vi "MAT Read Matrix.vi"(0 "Ref Num":refnum<file>, 5 "Error In":errorcluster) -> (6 "Matrix Name":string, 8 "Representation":T1, 9 "CSG":csg[][](array[numeric]) format="%.2f", 10 "STR":string[](array[string]), 11 "CDB":cdb[][](array[numeric]) format="%.2f", 12 "DBL":dbl[][](array[numeric]) format="%.2f", 13 "U8":u8[][](array[numeric]), 14 "Dup Ref Num":refnum<file>, 15 "SGL":sgl[][](array[numeric]) format="%.2f", 16 "I32":i32[][](array[numeric]), 17 "I16":i16[][](array[numeric]), 18 "U16":u16[][](array[numeric]), 19 "error out":errorcluster)   [LabVIEW 2013]
doc: "\"Save to MAT\" saves a 2D array of numbers or a 1D array of strings to MATLAB file. It works only with LabVIEW for Windows. All data types, described in MATLAB/External Interface Guide/Appendix A, are supported, except Sparse Matrices.\n\nAll data inputs should be 2D arrays, except String input which should be a 1D array. Only one data input may contain a non-empty array, otherwise error will be generated (error code -1).\n\nSAVML.LLB is a freeware written by Serge Liberman <liber@us1.channel1.com>."
uses:
  MAT Type Representation.ctl
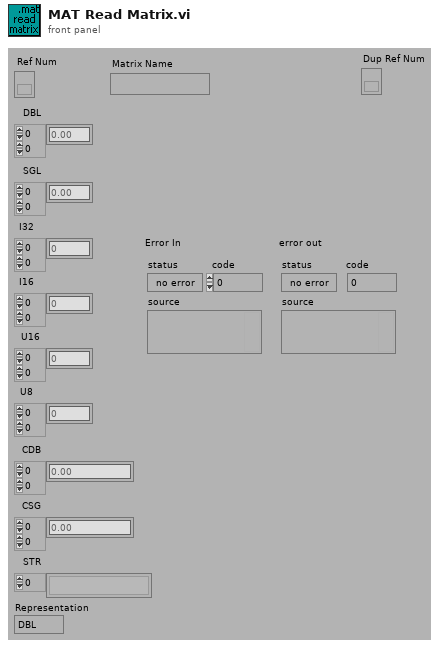
[diagram p1: front panel]
types:
  T1 = typedef "MAT Type Representation.ctl" = enum16{"DBL", "SGL", "I32", "I16", "U16", "U8", "CDB", "CSG", "STR"}
  T2 = enum16{"big-endian, network order", "native, host order", "little-endian"}
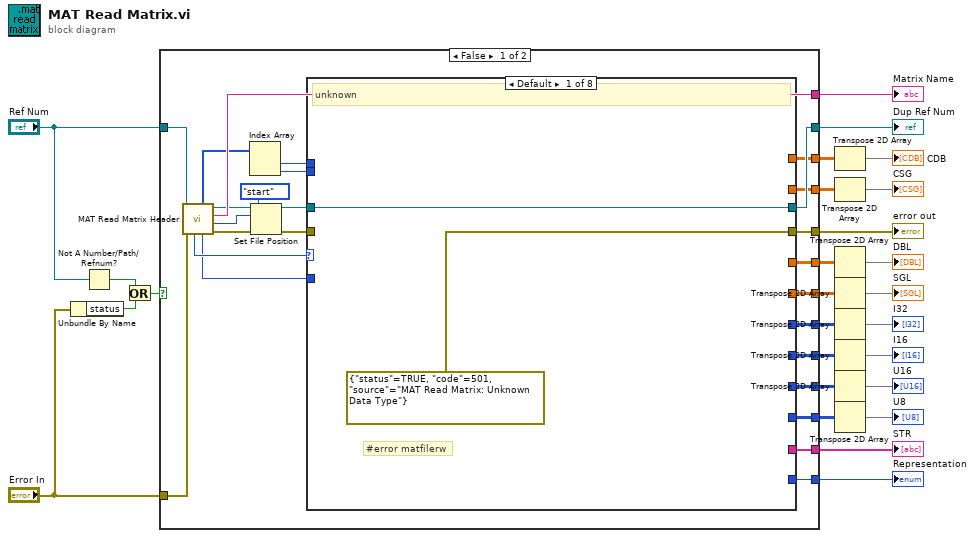
[diagram p0: block diagram]
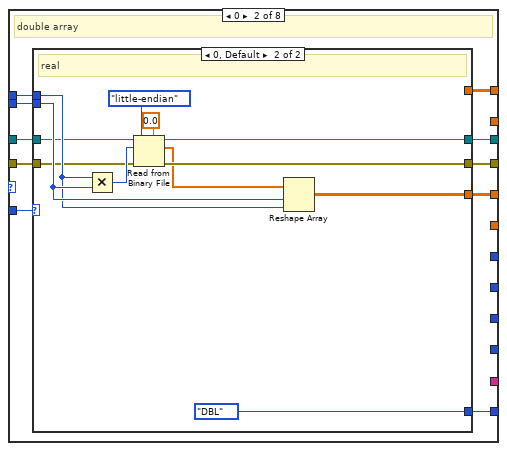
[diagram p2: hidden frame]
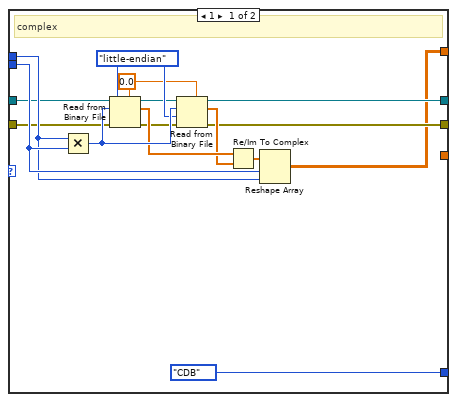
[diagram p3: hidden frame]
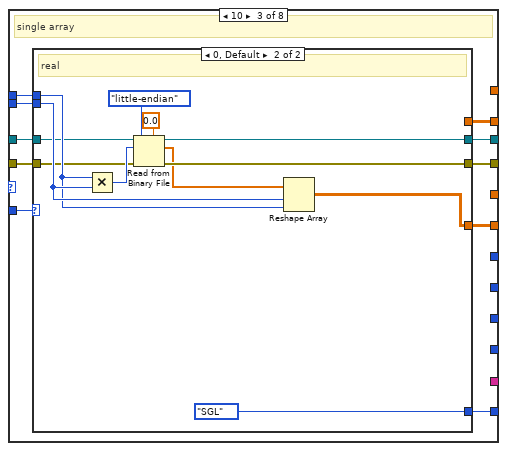
[diagram p4: hidden frame]
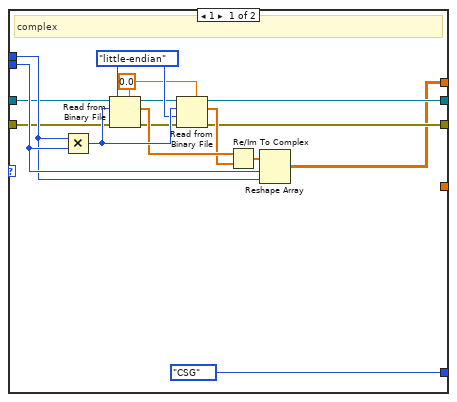
[diagram p5: hidden frame]
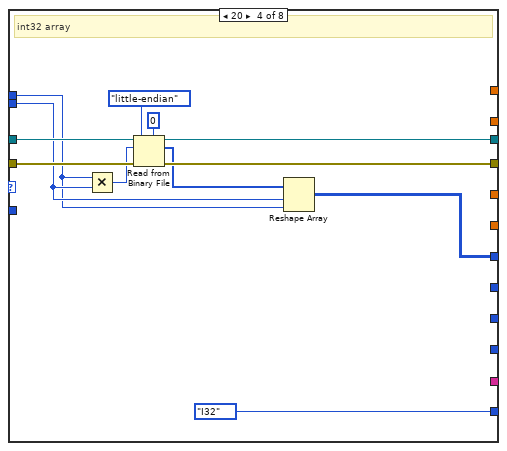
[diagram p6: hidden frame]
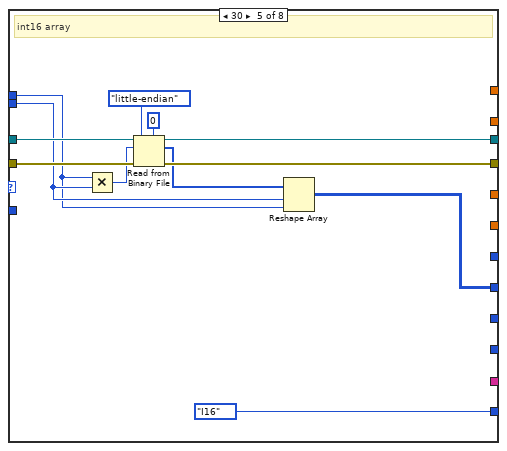
[diagram p7: hidden frame]
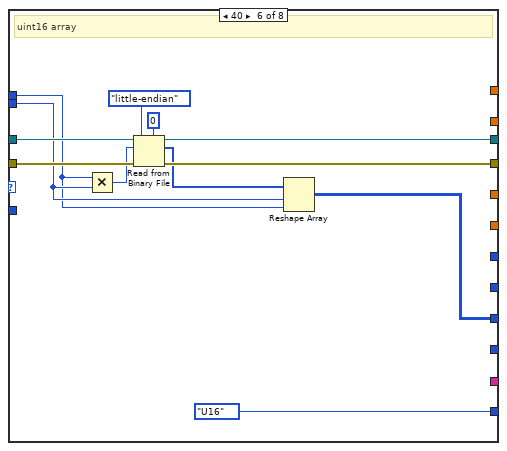
[diagram p8: hidden frame]
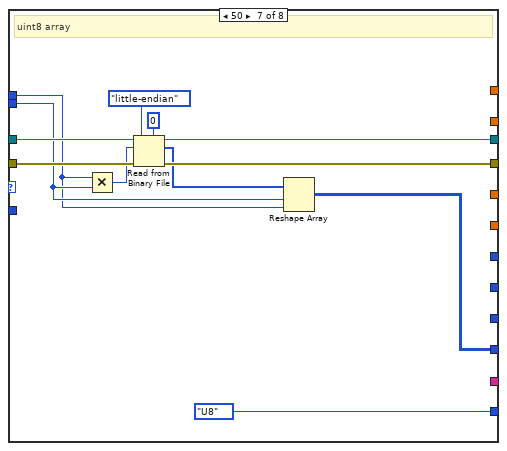
[diagram p9: hidden frame]
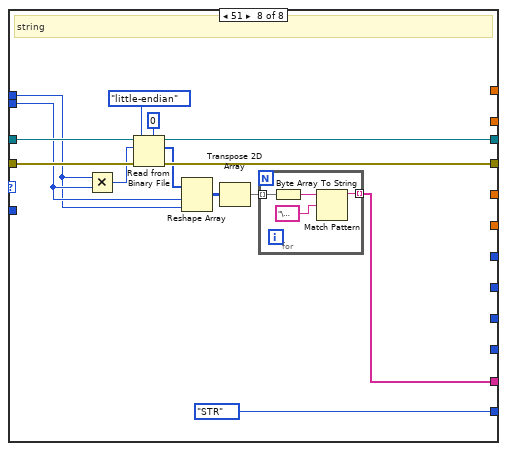
[diagram p10: hidden frame]
diagram:
  n1 = Unbundle By Name("Error In") -> ("status"=w23:bool)
  n2 = Not A Number/Path/Refnum?(number/path/refnum="Ref Num") -> (NaN/Path/Refnum?=w21:bool)
  n3 = Or(x=w21, y=w23) -> (x .or. y?=w20:bool)
  n4 = case shown="False" w20 {
    tunnel: [w52 w198] -> w26
    tunnel: "Ref Num" -> [w50 w198]
    tunnel: "Error In" -> [w36 w197]
    tunnel: [w51 w197] -> w24
    tunnel: [w48 _] -> w19
    tunnel: [w47 _] -> w18
    tunnel: [w46 _] -> w17
    tunnel: [w45 _] -> w16
    tunnel: [w43 _] -> w15
    tunnel: [w42 _] -> w14
    tunnel: [w41 _] -> w13
    tunnel: [w40 _] -> w12
    tunnel: [w39 _] -> w11
    tunnel: [w38 _] -> w3
    tunnel: [w37 _] -> w10
    frame False {
      n5 = call "MAT Read Matrix Header.vi"("Error In"=w36, "Ref Num"=w50) -> ("error out"=w31:errorcluster, "offset"=w29:i32, "Matrix Name"=w48:string, "Dup Ref Num"=w30:refnum<file>, "Real/Complex (0 - Real)"=w44:u32, "Matrix Size (rows x cols)"=w27:i32[], "Rep. Code"=w49:u32)  [unwired: 3 in]
      n6 = Index Array(array=w27) -> (element #1=w34:i32, element #2=w35:i32)  [unwired: 2 in]
      n7 = Set File Position(offset (in bytes) (0)=w29, refnum=w30, from (0:start)=enum16{"start", "end", "current"}."start", error in=w31) -> (refnum out=w32:refnum<file>, error out=w33:errorcluster)
      n8 = case shown="Default" w49 {
        tunnel: w32 -> [w54 w64 w102 w142 w154 w166 w178 w192]
        tunnel: [w54 w63 w101 w141 w153 w165 w177 w191] -> w52
        tunnel: w33 -> [_ w61 w99 w139 w151 w163 w175 w189]
        tunnel: [errorcluster {"status"=TRUE, "code"=501, "source"="MAT Read Matrix: Unknown Data Type"} ("error in (no error)") w62 w100 w140 w152 w164 w176 w190] -> w51
        tunnel: [_ w60 w98 MAT_Type_Representation."I32" ("Representation") MAT_Type_Representation."I16" ("Representation") MAT_Type_Representation."U16" ("Representation") MAT_Type_Representation."U8" ("Representation") MAT_Type_Representation."STR" ("Representation")] -> w47
        tunnel: w35 -> [_ w59 w97 w137 w149 w161 w173 w187]
        tunnel: w34 -> [_ w58 w96 w136 w148 w160 w172 w186]
        tunnel: [_ w57 _ _ _ _ _ _] -> w46
        tunnel: [_ _ w93 _ _ _ _ _] -> w45
        tunnel: w44 -> [_ w56 w95 _ _ _ _ _]
        tunnel: [_ _ _ w131 _ _ _ _] -> w43
        tunnel: [_ _ _ _ w143 _ _ _] -> w42
        tunnel: [_ _ _ _ _ w155 _ _] -> w41
        tunnel: [_ _ _ _ _ _ w167 _] -> w40
        tunnel: [_ _ _ _ _ _ _ w179] -> w39
        tunnel: [_ w55 _ _ _ _ _ _] -> w38
        tunnel: [_ _ w94 _ _ _ _ _] -> w37
        frame Default {
          # "#error matfilerw"
          # "unknown"
        }
        frame 0 {
          # "double array"
          n9 = case shown="0, Default" w56 {
            tunnel: w64 -> [w66 w85]
            tunnel: [w72 w83] -> w63
            tunnel: [w73 w84] -> w62
            tunnel: w61 -> [w67 w86]
            tunnel: [MAT_Type_Representation."CDB" ("Representation") MAT_Type_Representation."DBL" ("Representation")] -> w60
            tunnel: w59 -> [w71 w88]
            tunnel: w58 -> [w70 w87]
            tunnel: [_ w81] -> w57
            tunnel: [w65 _] -> w55
            frame 1 {
              w78 = T2."little-endian" ("byte order (0:big-endian, network order)")
              w77 = 0.0
              # "complex"
              n10 = Multiply(x=w70, y=w71) -> (x*y=w79:i32)
              n11 = Read from Binary File(5:w77, 8:w67, 9:w78, 10:w79, 11:w66) -> (0:w69:errorcluster, 2:w76:dbl[], 3:w68:refnum<file>)  [unwired: 1 in, 1 out]
              n12 = Read from Binary File(5:w77, 8:w69, 9:w78, 10:w79, 11:w68) -> (0:w73:errorcluster, 2:w75:dbl[], 3:w72:refnum<file>)  [unwired: 1 in, 1 out]
              n13 = Re/Im To Complex(1:w75, 2:w76) -> (0:w74:cdb[])
              n14 = Reshape Array(w74, w71, w70) -> (w65:cdb[][])
            }
            frame 0, Default {
              # "real"
              n15 = Multiply(x=w87, y=w88) -> (x*y=w91:i32)
              n16 = Read from Binary File(5:0.0, 8:w86, 9:T2."little-endian" ("byte order (0:big-endian, network order)"), 10:w91, 11:w85) -> (0:w84:errorcluster, 2:w82:dbl[], 3:w83:refnum<file>)  [unwired: 1 in, 1 out]
              n17 = Reshape Array(w82, w88, w87) -> (w81:dbl[][])
            }
          }
        }
        frame 10 {
          # "single array"
          n18 = case shown="0, Default" w95 {
            tunnel: w102 -> [w104 w123]
            tunnel: [w110 w121] -> w101
            tunnel: [w111 w122] -> w100
            tunnel: w99 -> [w105 w124]
            tunnel: [MAT_Type_Representation."CSG" ("Representation") MAT_Type_Representation."SGL" ("Representation")] -> w98
            tunnel: w97 -> [w109 w126]
            tunnel: w96 -> [w108 w125]
            tunnel: [w103 _] -> w94
            tunnel: [_ w119] -> w93
            frame 1 {
              w116 = T2."little-endian" ("byte order (0:big-endian, network order)")
              w115 = sgl 0.0
              # "complex"
              n19 = Multiply(x=w108, y=w109) -> (x*y=w117:i32)
              n20 = Read from Binary File(5:w115, 8:w105, 9:w116, 10:w117, 11:w104) -> (0:w107:errorcluster, 2:w114:sgl[], 3:w106:refnum<file>)  [unwired: 1 in, 1 out]
              n21 = Read from Binary File(5:w115, 8:w107, 9:w116, 10:w117, 11:w106) -> (0:w111:errorcluster, 2:w113:sgl[], 3:w110:refnum<file>)  [unwired: 1 in, 1 out]
              n22 = Re/Im To Complex(1:w113, 2:w114) -> (0:w112:csg[])
              n23 = Reshape Array(w112, w109, w108) -> (w103:csg[][])
            }
            frame 0, Default {
              # "real"
              n24 = Multiply(x=w125, y=w126) -> (x*y=w129:i32)
              n25 = Read from Binary File(5:sgl 0.0, 8:w124, 9:T2."little-endian" ("byte order (0:big-endian, network order)"), 10:w129, 11:w123) -> (0:w122:errorcluster, 2:w120:sgl[], 3:w121:refnum<file>)  [unwired: 1 in, 1 out]
              n26 = Reshape Array(w120, w126, w125) -> (w119:sgl[][])
            }
          }
        }
        frame 20 {
          # "int32 array"
          n27 = Multiply(x=w136, y=w137) -> (x*y=w135:i32)
          n28 = Read from Binary File(5:0, 8:w139, 9:T2."little-endian" ("byte order (0:big-endian, network order)"), 10:w135, 11:w142) -> (0:w140:errorcluster, 2:w132:i32[], 3:w141:refnum<file>)  [unwired: 1 in, 1 out]
          n29 = Reshape Array(w132, w137, w136) -> (w131:i32[][])
        }
        frame 30 {
          # "int16 array"
          n30 = Multiply(x=w148, y=w149) -> (x*y=w147:i32)
          n31 = Read from Binary File(5:i16 0, 8:w151, 9:T2."little-endian" ("byte order (0:big-endian, network order)"), 10:w147, 11:w154) -> (0:w152:errorcluster, 2:w144:i16[], 3:w153:refnum<file>)  [unwired: 1 in, 1 out]
          n32 = Reshape Array(w144, w149, w148) -> (w143:i16[][])
        }
        frame 40 {
          # "uint16 array"
          n33 = Multiply(x=w160, y=w161) -> (x*y=w159:i32)
          n34 = Read from Binary File(5:u16 0, 8:w163, 9:T2."little-endian" ("byte order (0:big-endian, network order)"), 10:w159, 11:w166) -> (0:w164:errorcluster, 2:w156:u16[], 3:w165:refnum<file>)  [unwired: 1 in, 1 out]
          n35 = Reshape Array(w156, w161, w160) -> (w155:u16[][])
        }
        frame 50 {
          # "uint8 array"
          n36 = Multiply(x=w172, y=w173) -> (x*y=w171:i32)
          n37 = Read from Binary File(5:u8 0, 8:w175, 9:T2."little-endian" ("byte order (0:big-endian, network order)"), 10:w171, 11:w178) -> (0:w176:errorcluster, 2:w168:u8[], 3:w177:refnum<file>)  [unwired: 1 in, 1 out]
          n38 = Reshape Array(w168, w173, w172) -> (w167:u8[][])
        }
        frame 51 {
          # "string"
          n39 = Multiply(x=w186, y=w187) -> (x*y=w185:i32)
          n40 = Read from Binary File(5:u8 0, 8:w189, 9:T2."little-endian" ("byte order (0:big-endian, network order)"), 10:w185, 11:w192) -> (0:w190:errorcluster, 2:w182:u8[], 3:w191:refnum<file>)  [unwired: 1 in, 1 out]
          n41 = Reshape Array(w182, w187, w186) -> (w181:u8[][])
          n42 = Transpose 2D Array(2D array=w181) -> (transposed array=w180:u8[][])
          n43 = for {
            tunnel: w180 -> [w196] mode=indexing
            tunnel: [w193] -> w179 mode=indexing
            n44 = Byte Array To String(unsigned byte array=w196) -> (string=w194:string)
            n45 = Match Pattern(string=w194, regular expression="\u0000") -> (before substring=w193:string)  [unwired: 1 in, 3 out]
          }
        }
      }
    }
    frame True {
    }
  }
  "error out" <- w24
  "Dup Ref Num" <- w26
  "Matrix Name" <- w19
  "Representation" <- w18
  "STR" <- w11
  n46 = Transpose 2D Array(2D array=w3) -> (transposed array=→"CDB":cdb[][])
  n47 = Transpose 2D Array(2D array=w10) -> (transposed array=→"CSG":csg[][])
  n48 = Transpose 2D Array(2D array=w17) -> (transposed array=→"DBL":dbl[][])
  n49 = Transpose 2D Array(2D array=w16) -> (transposed array=→"SGL":sgl[][])
  n50 = Transpose 2D Array(2D array=w15) -> (transposed array=→"I32":i32[][])
  n51 = Transpose 2D Array(2D array=w14) -> (transposed array=→"I16":i16[][])
  n52 = Transpose 2D Array(2D array=w13) -> (transposed array=→"U16":u16[][])
  n53 = Transpose 2D Array(2D array=w12) -> (transposed array=→"U8":u8[][])
